vi "Lakeshore 325 Test.vi"() -> ()   [LabVIEW 2022 SP3]
uses:
  <instrlib>/Lake Shore 325/Public/Data/Sensor Data (Single Reading).vi
  <instrlib>/Lake Shore 325/Lake Shore 325.lvlib
panel:
  out "error out":errorcluster
  out "Sensor Data":dbl format="%.4f"
  in  "Serial Configuration":T1={"Baud Rate"=9600, "Parity"=1, "Data Bits"=7, "Stop Bits"=10, "Flow Control"=0} {"Flow Control" items=["None", "XON/XOFF", "RTS/CTS", "XON/XOFF & RTS/CTS", "DTR/DSR", "XON/XOFF & DTR/DSR"]; "Stop Bits" items=["1.0"=10, "1.5"=15, "2.0"=20]; "Data Bits" items=["7"=7, "8"=8]; "Parity" items=["None", "Odd", "Even", "Mark", "Space"]; "Baud Rate" items=["300"=300, "600"=600, "1200"=1200, "2400"=2400, "4800"=4800, "9600"=9600, "19200"=19200, "38400"=38400, "57600"=57600]}
  in  "VISA resource name":refnum<visa-resource-name>="GPIB0::12::INSTR"
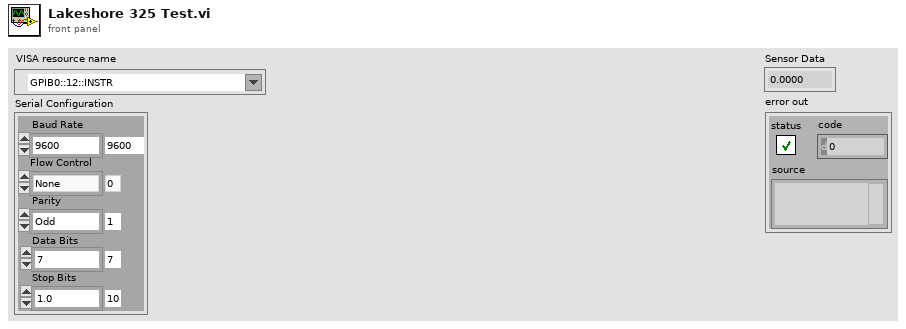
[diagram p1: front panel]
types:
  T1 = cluster{"Baud Rate":u32, "Parity":u16, "Data Bits":u16, "Stop Bits":u16, "Flow Control":u16}
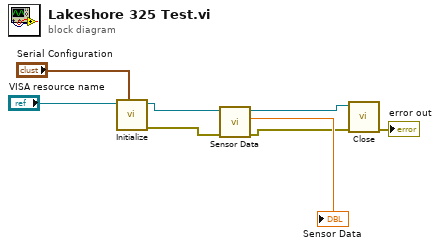
[diagram p0: block diagram]
diagram:
  n1 = call <instrlib>:"Initialize.vi"("Serial Configuration"="Serial Configuration", "VISA resource name"="VISA resource name") -> ("error out"=w3:errorcluster, "VISA resource name out"=w8:refnum<visa-resource-name>)  [unwired: 8 in]
  n2 = call-poly <instrlib>:"Sensor Data.vi"("error in (no error)"=w3, "VISA resource name"=w8) -> ("error out"=w2:errorcluster, "Sensor Data"=→"Sensor Data":dbl, "VISA resource name out"=w4:refnum<visa-resource-name>)  [unwired: 7 in]
  n3 = call <instrlib>:"Close.vi"("error in (no error)"=w2, "VISA resource name"=w4) -> ("error out"=→"error out":errorcluster)  [unwired: 9 in]
